vi "STAV Write_read.vi"(6 "delay (20)":u32=20, 8 "error in (no error)":errorcluster, 10 "Str cmd":string, 11 "STAV ref in":refnum<visa-resource-name>) -> (0 "error out":errorcluster, 2 "Str out":string, 3 "STAV ref out":refnum<visa-resource-name>)   [LabVIEW 2021, in "STAV lib.lvlib"]
doc: "Write command to device, wait a delay time and reads answer"
uses:
  STAV lib.lvlib
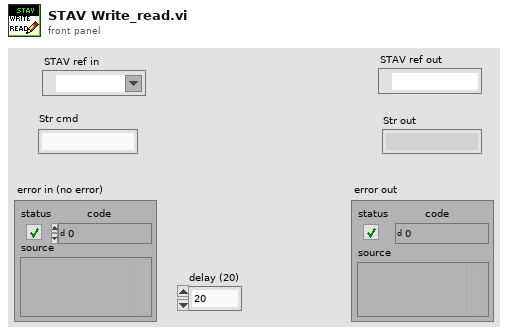
[diagram p1: front panel]
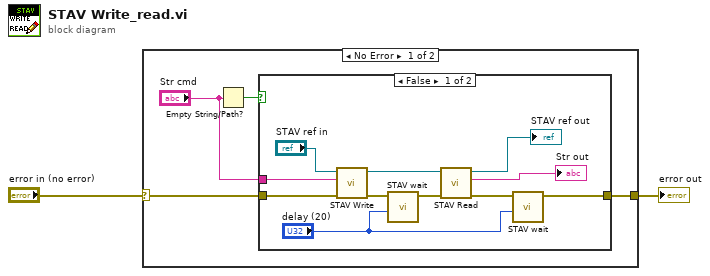
[diagram p0: block diagram]
diagram:
  n1 = case shown="No Error" "error in (no error)" {
    selector: "error in (no error)" -> [w5 w19]
    tunnel: [w3 w19] -> w1
    frame No Error {
      n2 = Empty String/Path?(string/path="Str cmd") -> (empty?=w6:bool)
      n3 = case shown="False" w6 {
        tunnel: w5 -> [w16 w18]
        tunnel: "Str cmd" -> [w14 _]
        tunnel: [w9 w18] -> w3
        frame False {
          n4 = call "STAV Write.vi"("error in (no error)"=w16, "Command"=w14, "STAV ref in"="STAV ref in") -> ("error out"=w17:errorcluster, "STAV ref out"=w12:refnum<visa-resource-name>)  [unwired: 7 in]
          n5 = call "STAV wait.vi"("delay (20)"="delay (20)", "error in (no error)"=w17) -> ("error out"=w15:errorcluster)  [unwired: 9 in]
          n6 = call "STAV Read.vi"("error in (no error)"=w15, "STAV ref in"=w12) -> ("error out"=w10:errorcluster, "String"=→"Str out":string, "STAV ref out"=→"STAV ref out":refnum<visa-resource-name>)  [unwired: 6 in, 1 out]
          n7 = call "STAV wait.vi"("delay (20)"="delay (20)", "error in (no error)"=w10) -> ("error out"=w9:errorcluster)  [unwired: 9 in]
        }
        frame True {
        }
      }
    }
    frame Error {
    }
  }
  "error out" <- w1
